vi "Main.vi"() -> ()   [LabVIEW 2022 SP3]
panel:
  in  "Enter for interferecese":bool
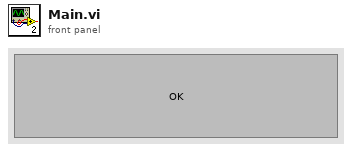
[diagram p1: front panel]
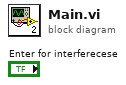
[diagram p0: block diagram]
diagram:
